vi "$TEST_TankControl18V7.vi"(11 "Inputs":T1={"Fill!Drain"=TRUE, "Speed"=2, "Send Msg"=FALSE, "Write Buf"="GO"} {"Speed" scale=0.0..100.0}) -> (2 "Laser Raw":sgl=2.4953, 3 "Outputs":T3={"Status"=[TRUE, FALSE, FALSE, FALSE, FALSE, FALSE, FALSE, FALSE, FALSE, FALSE, FALSE, FALSE, FALSE, FALSE, FALSE, FALSE, FALSE, FALSE, FALSE, FALSE, FALSE, FALSE, FALSE, FALSE, FALSE, FALSE, FALSE, FALSE, FALSE, FALSE, FALSE, FALSE], "Match"=-1, "Rx Speed"=".+64", "Tx"=FALSE})   [LabVIEW 2024]
uses:
  Control Definitions/Def_Status18v7.ctl
  <instrlib>/Keyence LK-G3000/Keyence LK-G3000.lvlib
panel:
  out "Elapsed":dbl format="%#.2g"
  out "Rate In/Min":dbl=nan format="%#.4g"
  in  "Reset":bool
  in  "Start":bool
  in  "Time (sec)":dbl=30.0
  in  "Laser ON":bool=TRUE
  out "Level PV":dbl(slide)=7.1220598220825195 scale=0.0..10.0
  in  "Send Reply":bool
  out "TX Buf":string="D0\r"
  in  "Send Reply Buf":string
  out "read buffer ASC":string="!1\r\n"
  in  "Exit":bool
  # "Use this Timer section\nto measure the Level dl/dt"
  # "Laser ON When Laser\nis on Line."
  # "Use if off line to generate\na test Reply to Write msg"
  # "Target Speed for PWC OLS = 0.52\"/min\nWhich is Speed set to ~17% which 24Vdc"
  # "Fill"
  # "Drain"
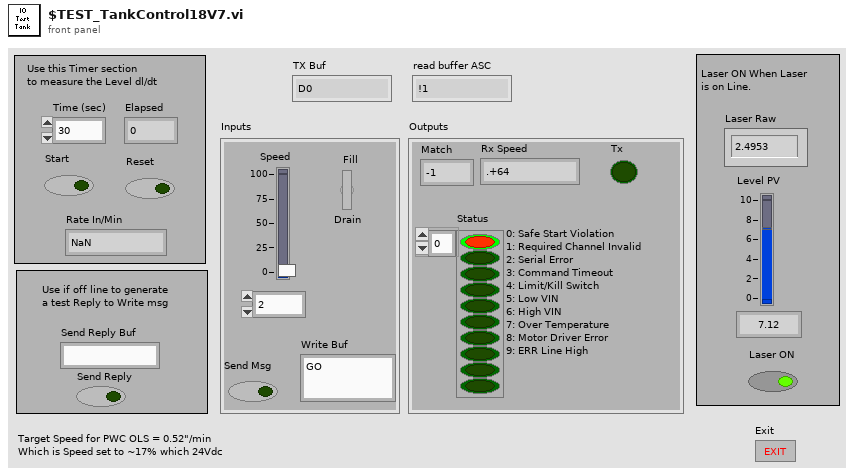
[diagram p1: front panel]
types:
  T1 = cluster{"Fill!Drain":bool, "Speed":i16, "Send Msg":bool, "Write Buf":string}
  T2 = typedef "Def_Status18v7.ctl" = bool[]
  T3 = cluster{"Status":T2, "Match":i32, "Rx Speed":string, "Tx":bool}
  T4 = typedef "Keyence LK-G3000.lvlib/LKIF_FLOATVALUE.ctl" = cluster{"LKIF_FLOATRESULT":T5, "Value":sgl}
  T5 = typedef "Keyence LK-G3000.lvlib/LKIF_FLOATRESULT.ctl" = i32
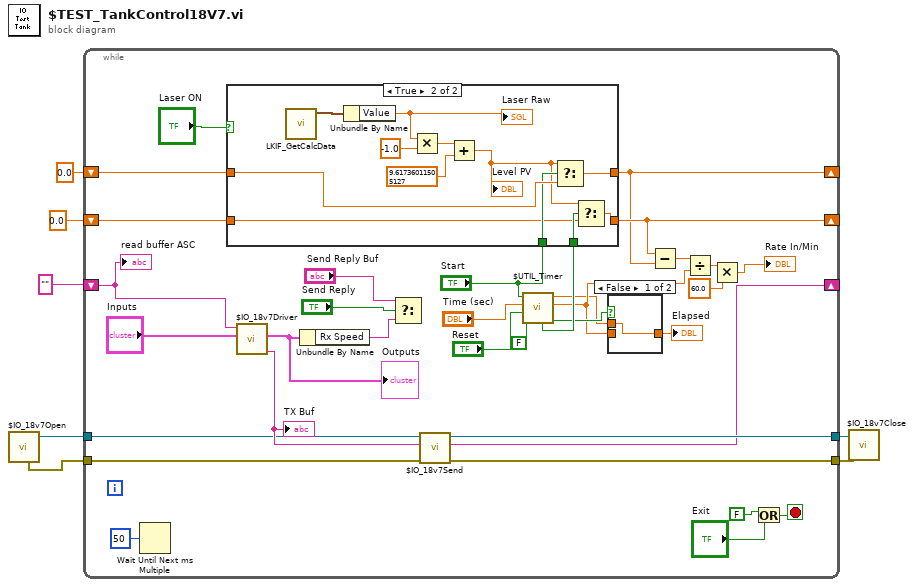
[diagram p0: block diagram]
diagram:
  n1 = call "$IO_18v7Open.vi"() -> ("VISA Refnum out"=w6:refnum<visa-resource-name>, "error out"=w1:errorcluster)  [unwired: 9 in, 1 out]
  n2 = while {
    shift-right: [w28] -> _
    shift-left: "" ("Repy") -> [w34]
    tunnel: w6 -> [w30]
    tunnel: [w29] -> w5
    shift-right: [w19] -> _
    shift-left: sgl 0.0 -> [w26]
    shift-right: [w20] -> _
    shift-left: sgl 0.0 -> [w22]
    tunnel: w1 -> [w12]
    tunnel: [w11] -> w2
    stop <- w41 stop-if-true
    n3 = Wait Until Next ms Multiple(millisecond multiple=u32 50) -> ()  [unwired: 1 out]
    n4 = call "$IO_18v7Driver.vi"("Inputs"="Inputs", "Reply In"=w34) -> ("Tx Buf Out"=w31:string, "Outputs"=w33:T3)  [unwired: 8 in]
    "TX Buf" <- w31
    "Outputs" <- w33
    n5 = Unbundle By Name(w33) -> ("Rx Speed"=w32:string)
    n6 = Select(t="Send Reply Buf", s="Send Reply", f=w32) -> ()  [unwired: 1 out]
    n7 = call "$IO_18v7Send.vi"("error in (no error)"=w12, "Tx Buf Out"=w31, "VISA Refnum in"=w30) -> ("error out"=w11:errorcluster, "read buffer"=w28:string, "VISA Refnum out"=w29:refnum<visa-resource-name>)  [unwired: 6 in]
    n8 = call "$UTIL_Timer.vi"("Auto Reset"=FALSE, "Reset"="Reset", "Time (sec)"="Time (sec)", "Start"="Start") -> ("Timed Out"=w16:bool, "Numeric 2"=w15:dbl, "Elapsed"=w13:dbl, "TO Trig"=w21:bool)  [unwired: 2 in, 2 out]
    n9 = case shown="True" "Laser ON" {
      tunnel: [w45 w52] -> w19
      tunnel: w26 -> [w45 w51]
      tunnel: "Start" -> [_ w50]
      tunnel: w21 -> [_ w49]
      tunnel: [w44 w48] -> w20
      tunnel: w22 -> [w44 w47]
      frame False {
      }
      frame True {
        n10 = call <instrlib>:"LKIF_GetCalcData.vi"() -> ("CalcData1"=w57:T4)  [unwired: 9 in, 2 out]
        n11 = Unbundle By Name(w57) -> ("Value"=w56:sgl)
        "Laser Raw" <- w56
        n12 = Multiply(x=w56, y=sgl -1.0) -> (x*y=w54:sgl)
        n13 = Add(x=w54, y=sgl 9.61736) -> (x+y=w46:sgl)
        "Level PV" <- w46
        n14 = Select(t=w46, s=w50, f=w51) -> (s? t:f=w52:sgl)
        n15 = Select(t=w46, s=w49, f=w47) -> (s? t:f=w48:sgl)
      }
    }
    n16 = case shown="False" w16 {
      tunnel: w15 -> [_ w43]
      tunnel: [w42 w43] -> w14
      tunnel: w13 -> [w42 _]
      frame False {
      }
      frame True {
      }
    }
    "Elapsed" <- w14
    n17 = Subtract(x=w20, y=w19) -> (x-y=w18:sgl)
    n18 = Divide(x=w18, y=w15) -> (x/y=w10:dbl)
    n19 = Multiply(x=w10, y=60.0) -> (x*y=→"Rate In/Min":dbl)
    n20 = Or(x=FALSE, y="Exit") -> (x .or. y?=w41:bool)
    "read buffer ASC" <- w34
  }
  n21 = call "$IO_18v7Close.vi"("error in (no error)"=w2, "VISA Refnum in"=w5) -> ()  [unwired: 10 in]
